vi "Write.vi"   [LabVIEW 2014, in "LMH-LINX.lvlib" / "WS2812.lvlib"]
uses:
  <vilib>/MakerHub/LINX/Public/Sensors/Lights/WS2812/WS2812.lvlib
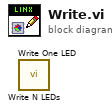
[diagram p0: block diagram]
diagram:
  n1 = call <vilib>:"Write N LEDs.vi"() -> ()  [unwired: 10 in, 2 out]
  n2 = call <vilib>:"Write One LED.vi"() -> ()  [unwired: 10 in, 2 out]
